vi "Insert Start Message.vi"(8 "error in (no error)":errorcluster, 10 "Start Time":timestamp, 11 "AcquireTraces in":refnum<class "AcquireTraces.lvclass">) -> (0 "error out":errorcluster, 3 "AcquireTraces out":refnum<class "AcquireTraces.lvclass">)   [LabVIEW 2011, in "AcquireTraces.lvclass"]
uses:
  AcquireTraces.lvclass
  AcquistionObject/AcquistionObject.lvclass
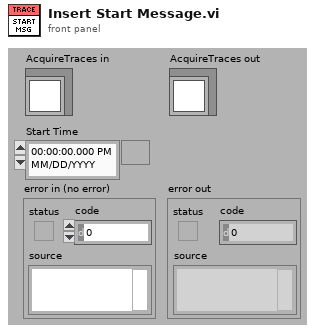
[diagram p1: front panel]
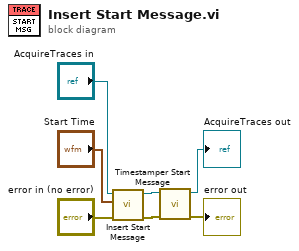
[diagram p0: block diagram]
diagram:
  n1 = call-parent "Insert Start Message.vi"("error in (no error)"="error in (no error)", "Start Time"="Start Time", "AcquistionObject in"="AcquireTraces in") -> ("error out"=w3:errorcluster, "AcquistionObject out"=w4:refnum<class "AcquireTraces.lvclass">)  [unwired: 7 in]
  n2 = call-dynamic "Timestamper Start Message.vi"("error in (no error)"=w3, "AcquistionObject in"=w4) -> ("error out"=→"error out":errorcluster, "AcquistionObject out"=→"AcquireTraces out":refnum<class "AcquireTraces.lvclass">)  [unwired: 8 in]
